vi "CoordinateDataEntry.vi"(7 "CoordinateAction":T12, 8 "error in (no error)":errorcluster, 11 "OneCoordStep Input":T1={"ProcessSetting"=[], "Project Name"="Pattern", "AnalysisSetting"=[], "Coord?"=FALSE, "OriginPointInfo"={"Output Original"=FALSE, "Origin Name"="", "Angle"=0.0, "Mode"=0, "OriginPoint"={"X"=0.0, "Y"=0.0}}, "CaliperSetting"=[], "CoordIndex"=[]} {"CaliperSetting"."CaliperEntry"."CaliperType" items=["Distance", "Mid Point", "Perpendicular Projection", "Lines Intersection", "Angle from Horizontal", "Angle from Vertical", "Angle Defined by 3 Points", "Angle Defined by 4 Points", "Bissecting Line", "Mid Line", "Center of Mass", "Area", "Line Fit", "Circle Fit", "Ellipse Fit"]; "OriginPointInfo"."Mode" items=["Horizontal Motion", "Vertical Motion", "Horizontal and Vertical Motion", "Horizontal. Vertical and Angular Motion"]; "AnalysisSetting"."ROI"."Contours"."Type" items=["No Selection", "Point", "Line", "Rectangle", "Oval", "Polygon", "Freehand Region", "Annulus", "Unused2", "Unused3", "Broken Line", "Freehand Line", "Rotated Rectangle"]}) -> (0 "error out":errorcluster, 3 "CoordinatteEntry Output":T1={"ProcessSetting"=[], "Project Name"="Pattern", "AnalysisSetting"=[], "Coord?"=FALSE, "OriginPointInfo"={"Output Original"=FALSE, "Origin Name"="", "Angle"=0.0, "Mode"=0, "OriginPoint"={"X"=0.0, "Y"=0.0}}, "CaliperSetting"=[], "CoordIndex"=[]} {"CaliperSetting"."CaliperEntry"."CaliperType" items=["Distance", "Mid Point", "Perpendicular Projection", "Lines Intersection", "Angle from Horizontal", "Angle from Vertical", "Angle Defined by 3 Points", "Angle Defined by 4 Points", "Bissecting Line", "Mid Line", "Center of Mass", "Area", "Line Fit", "Circle Fit", "Ellipse Fit"]; "OriginPointInfo"."Mode" items=["Horizontal Motion", "Vertical Motion", "Horizontal and Vertical Motion", "Horizontal. Vertical and Angular Motion"]; "AnalysisSetting"."ROI"."Contours"."Type" items=["No Selection", "Point", "Line", "Rectangle", "Oval", "Polygon", "Freehand Region", "Annulus", "Unused2", "Unused3", "Broken Line", "Freehand Line", "Rotated Rectangle"]})   [LabVIEW 2015]
uses:
  Control/CoordinateAction.ctl
  Control/CoordinatteEntry.ctl
  Process/Controls/Process_Setting.ctl
  Process/Controls/Process_Type.ctl
  Control/CoordinateAnalysisSetting.ctl
  Control/CoordinateCaliperSetting.ctl
  Caliper/Controls/CaliperDataEntry.ctl
  Caliper/Controls/CaliperType.ctl
  Caliper/Controls/SelectionListEntry.ctl
  Caliper/Controls/SelectionListEntryPointType.ctl
  Caliper/Controls/CaliperResult.ctl
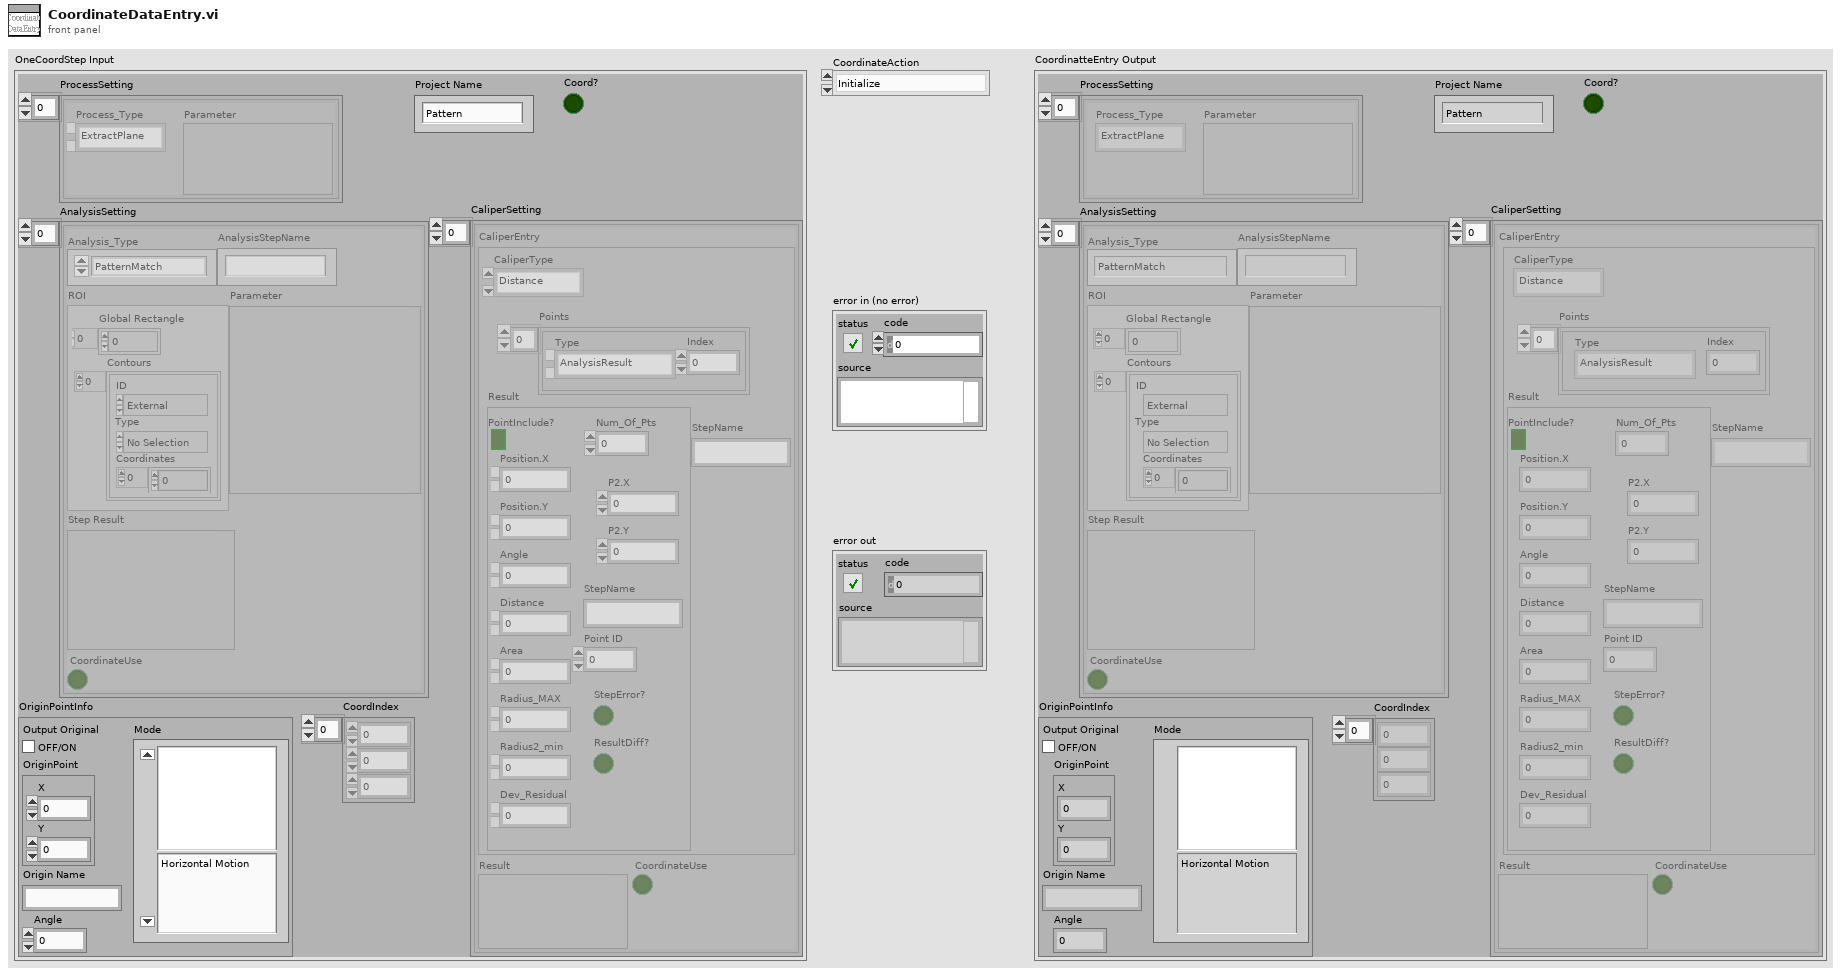
[diagram p1: front panel]
types:
  T1 = typedef "CoordinatteEntry.ctl" = cluster{"ProcessSetting":T2[], "Project Name":string, "AnalysisSetting":T4[], "Coord?":bool, "OriginPointInfo":cluster{"Output Original":bool, "Origin Name":string, "Angle":dbl, "Mode":u16, "OriginPoint":cluster{"X":dbl, "Y":dbl}}, "CaliperSetting":T6[], "CoordIndex":i32[]}
  T2 = typedef "Process_Setting.ctl" = cluster{"Process_Type":T3, "Parameter":variant}
  T3 = typedef "Process_Type.ctl" = enum16{"None", "ExtractPlane", "BinaryMono", "Operators", "GrayMorphology", "Filters", "Lookup Table", "Particle Filter", "Mask"}
  T4 = typedef "CoordinateAnalysisSetting.ctl" = cluster{"Analysis_Type":enum16{"PatternMatch", "Straight Edge"}, "ROI ":T5, "Parameter":variant, "Step Result":variant, "AnalysisStepName":string, "CoordinateUse":bool}
  T5 = typedef "ROI Descriptor" = cluster{"Global Rectangle":i32[], "Contours":cluster{"ID":enum32{"External", "Internal"}, "Type":u32, "Coordinates":i32[]}[]}
  T6 = typedef "CoordinateCaliperSetting.ctl" = cluster{"Result":variant, "CoordinateUse":bool, "CaliperEntry":T7}
  T7 = typedef "CaliperDataEntry.ctl" = cluster{"CaliperType":T8, "Points":T9[], "Result":T11, "StepName":string}
  T8 = typedef "CaliperType.ctl" = u32
  T9 = typedef "SelectionListEntry.ctl" = cluster{"Type":T10, "Index":i32}
  T10 = typedef "SelectionListEntryPointType.ctl" = enum16{"AnalysisResult", "CaliperResult"}
  T11 = typedef "CaliperResult.ctl" = cluster{"PointInclude?":bool, "Num_Of_Pts":u8, "Position.X":dbl, "Position.Y":dbl, "Angle":dbl, "Distance":dbl, "Area":dbl, "Radius_MAX":dbl, "Radius2_min":dbl, "Dev_Residual":dbl, "P2.X":dbl, "P2.Y":dbl, "StepName":string, "Point ID":u8, "StepError?":bool, "ResultDiff?":bool}
  T12 = typedef "CoordinateAction.ctl" = enum16{"Initialize", "CoordEntryInput", "CoordEntryOutput", "CoordEntryTemp", "CoordEntryBackup", "CoordEntryReturn"}
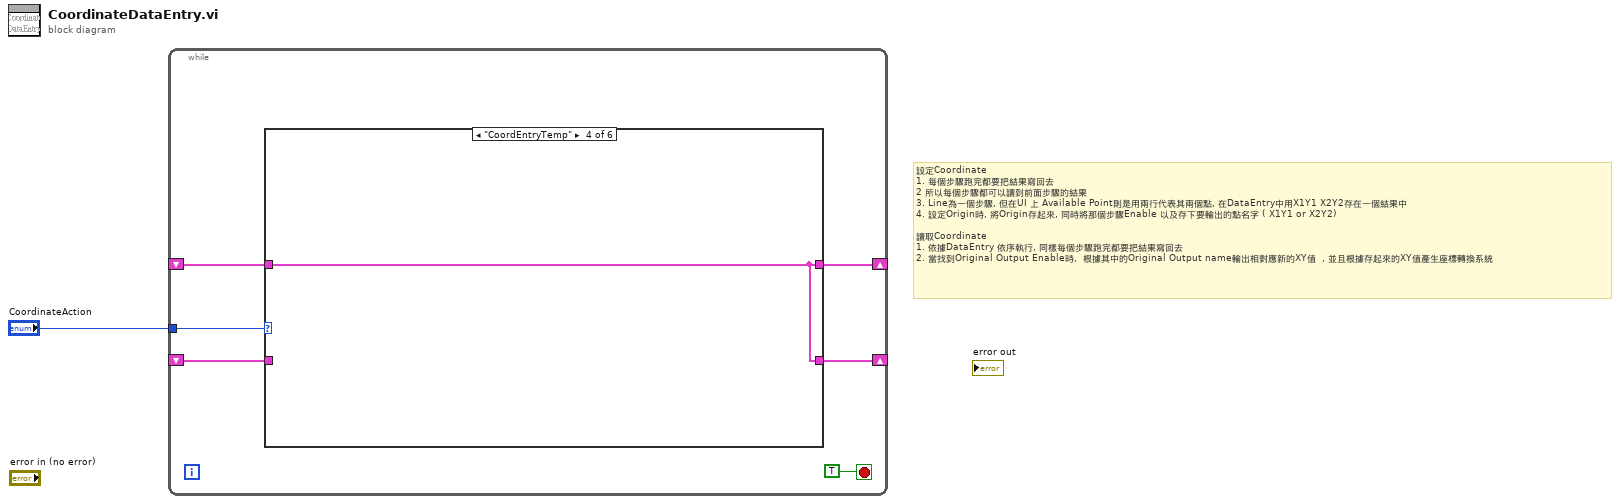
[diagram p0: block diagram]
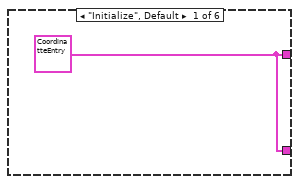
[diagram p2: hidden frame]
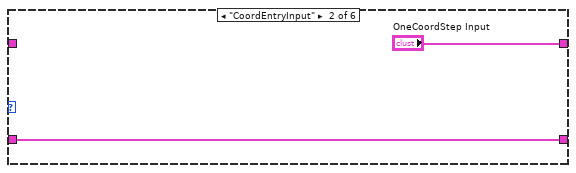
[diagram p3: hidden frame]
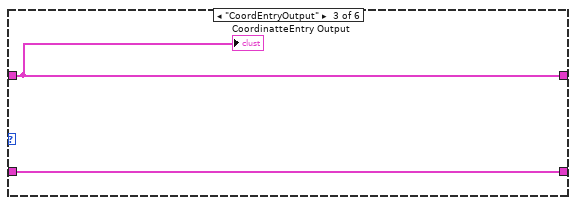
[diagram p4: hidden frame]
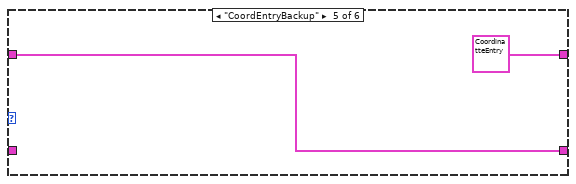
[diagram p5: hidden frame]
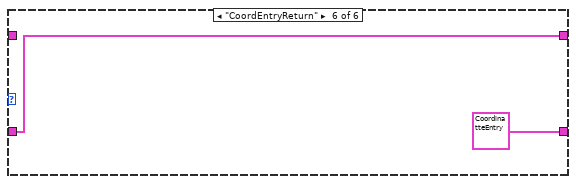
[diagram p6: hidden frame]
diagram:
  # "設定Coordinate\n1. 每個步驟跑完都要把結果寫回去\n2 所以每個步驟都可以讀到前面步驟的結果\n3. Line為一個步驟, 但在UI 上 Available Point則是用兩行代表其兩個點, 在DataEntry中用X1Y1 X2Y2存在一個結果中\n4. 設定Origin時, 將Origin存起來, 同時將那個步驟Enable 以及存下要輸出的點名字 ( X1Y1 or X2Y2)\n\n讀取Coordinate\n1. 依據DataEntry 依序執行, 同樣每個步驟跑完都要把結果寫回去\n2. 當找到Original Output Enable時,  根據其中的Original Output name輸出相對應新的XY值  , 並且根據存起來的XY值產生座標轉換系統"
  n1 = while {
    tunnel: "CoordinateAction" -> [w7]
    shift-right: [w6] -> _
    shift-left: _ -> [w5]
    shift-right: [w3] -> _
    shift-left: _ -> [w2]
    stop <- TRUE stop-if-true
    n2 = case shown="\"CoordEntryTemp\"" w7 {
      tunnel: [w8 "OneCoordStep Input" w12 w13 T1 {"ProcessSetting"=[], "Project Name"="", "AnalysisSetting"=[], "Coord?"=FALSE, "OriginPointInfo"={"Output Original"=FALSE, "Origin Name"="", "Angle"=0.0, "Mode"=0, "OriginPoint"={"X"=0.0, "Y"=0.0}}, "CaliperSetting"=[], "CoordIndex"=[]} ("OneCoordStep Input") w17] -> w6
      tunnel: w5 -> [_ _ w12 w13 w15 _]
      tunnel: [w8 w9 w11 w13 w15 T1 {"ProcessSetting"=[], "Project Name"="", "AnalysisSetting"=[], "Coord?"=FALSE, "OriginPointInfo"={"Output Original"=FALSE, "Origin Name"="", "Angle"=0.0, "Mode"=0, "OriginPoint"={"X"=0.0, "Y"=0.0}}, "CaliperSetting"=[], "CoordIndex"=[]} ("OneCoordStep Input")] -> w3
      tunnel: w2 -> [_ w9 w11 _ _ w17]
      frame "Initialize", Default {
        w8 = T1 {"ProcessSetting"=[], "Project Name"="", "AnalysisSetting"=[], "Coord?"=FALSE, "OriginPointInfo"={"Output Original"=FALSE, "Origin Name"="", "Angle"=0.0, "Mode"=0, "OriginPoint"={"X"=0.0, "Y"=0.0}}, "CaliperSetting"=[], "CoordIndex"=[]} ("OneCoordStep Input")
      }
      frame "CoordEntryInput" {
      }
      frame "CoordEntryOutput" {
        "CoordinatteEntry Output" <- w12
      }
      frame "CoordEntryTemp" {
      }
      frame "CoordEntryBackup" {
      }
      frame "CoordEntryReturn" {
      }
    }
  }
